vi "Write Queue Ref.vi"(8 "error in":errorcluster, 10 "Queue Ref":refnum<queue>, 11 "QueueMessageTransport in":refnum<class "QueueMessageTransport.lvclass">) -> (0 "error out":errorcluster, 3 "QueueMessageTransport out":refnum<class "QueueMessageTransport.lvclass">)   [LabVIEW 2016, in "QueueMessageTransport.lvclass"]
uses:
  QueueMessageTransport.lvclass
  IMessagePayload/IMessagePayload.lvclass
  QueueMessageTransport.lvclass/QueueMessageTransport.ctl
panel:
  # "INPUTS"
  # "OUTPUTS"
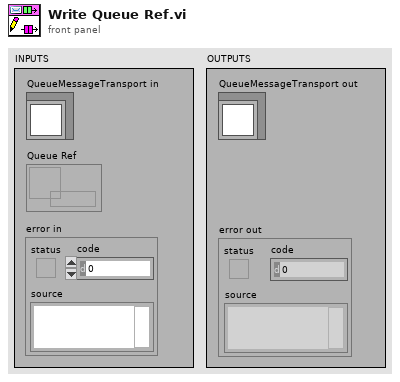
[diagram p1: front panel]
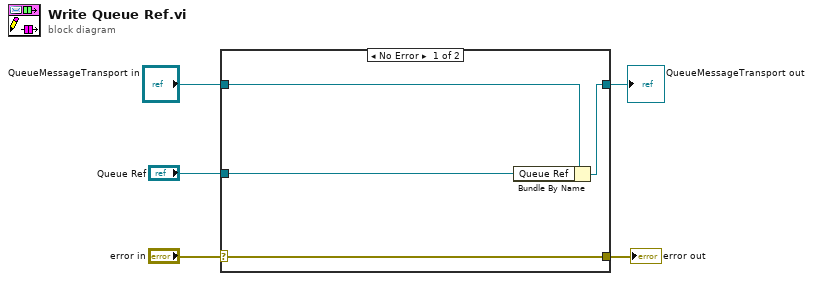
[diagram p0: block diagram]
diagram:
  n1 = case shown="No Error" "error in" {
    selector: "error in" -> [w9 w10]
    tunnel: [w9 w10] -> w4
    tunnel: [w7 w11] -> w2
    tunnel: "QueueMessageTransport in" -> [w8 w11]
    tunnel: "Queue Ref" -> [w6 _]
    frame No Error {
      n2 = Bundle By Name(cluster=w8, "Queue Ref"=w6) -> (w7:refnum<class "QueueMessageTransport.lvclass">)
    }
    frame Error {
    }
  }
  "error out" <- w4
  "QueueMessageTransport out" <- w2
